vi "Set RX Data Width.vi"(8 "error in":errorcluster, 10 "rx internal data width":T1=enum."32 Bit", 11 "eye scan in":refnum<class "niHighSpeedSerial Eye Scan v1 Host.lvclass">) -> (0 "error out":errorcluster, 3 "eye scan out":refnum<class "niHighSpeedSerial Eye Scan v1 Host.lvclass">)   [LabVIEW 2015, in "niHighSpeedSerial Eye Scan v1 Host.lvclass"]
uses:
  <instrlib>/niHighSpeedSerial/Eye Scan/v1/Host/Eye Scan/niHighSpeedSerial Eye Scan v1 Host.lvclass
  <instrlib>/niHighSpeedSerial/Eye Scan/v1/Host/Common/Public/Data Width.ctl
  <instrlib>/niHighSpeedSerial/Eye Scan/v1/Host/Eye Scan/niHighSpeedSerial Eye Scan v1 Host.lvclass/niHighSpeedSerial Eye Scan v1 Host.ctl
  <vilib>/Utility/error.llb/Error Cluster From Error Code.vi
  <vilib>/ErrorRing/Error Ring.xnode
  <instrlib>/niHighSpeedSerial/Eye Scan/v1/Host/Common/niHighSpeedSerial Eye Scan Common v1 Host.lvlib
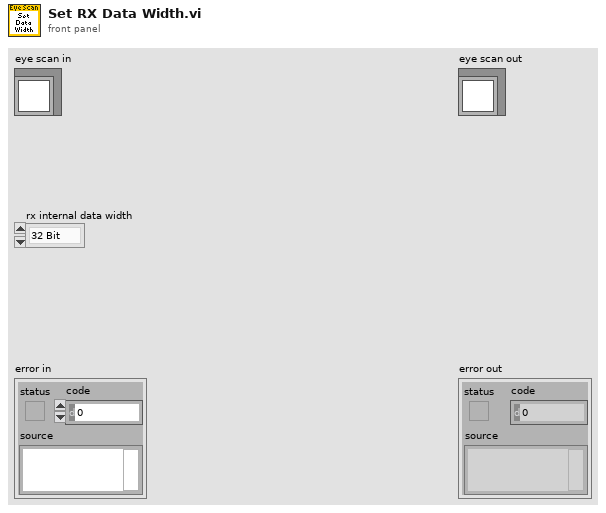
[diagram p1: front panel]
types:
  T1 = typedef "niHighSpeedSerial Eye Scan Common v1 Host.lvlib/Data Width.ctl" = enum16{"16 Bit", "20 Bit", "32 Bit", "40 Bit"}
  T2 = typedef "niHighSpeedSerial Eye Scan v1 Host.lvclass/Private Data.ctl" = cluster{"instruction target":refnum<class "niInstr Instruction Target v1 Host.lvclass">, "channels":T3[], "measure state":T4, "rx output divider":T5, "equalization mode":T6, "rx internal data width":T1, "BER floor":dbl, "number of points completed":i32, "rx output divider configured?":bool, "equalization mode configured?":bool, "rx data width configured?":bool}
  T3 = typedef "niHighSpeedSerial Eye Scan v1 Host.lvclass/Channel Data.ctl" = cluster{"instance":u8, "channel":refnum<class "niHighSpeedSerial Eye Scan Single Point v1 Host.lvclass">, "point iterator":refnum<class "niHighSpeedSerial Eye Scan Point Iterator v1 Host.lvclass">}
  T4 = typedef "niHighSpeedSerial Eye Scan v1 Host.lvclass/Measure State.ctl" = enum16{"Uninitialized", "Initialized", "Ready", "Measuring", "Finished", "Aborted"}
  T5 = typedef "niHighSpeedSerial Eye Scan Common v1 Host.lvlib/RX Output Divider.ctl" = enum16{"1", "2", "4", "8", "16"}
  T6 = typedef "niHighSpeedSerial Eye Scan Common v1 Host.lvlib/Equalization Mode.ctl" = enum16{"DFE", "LPM"}
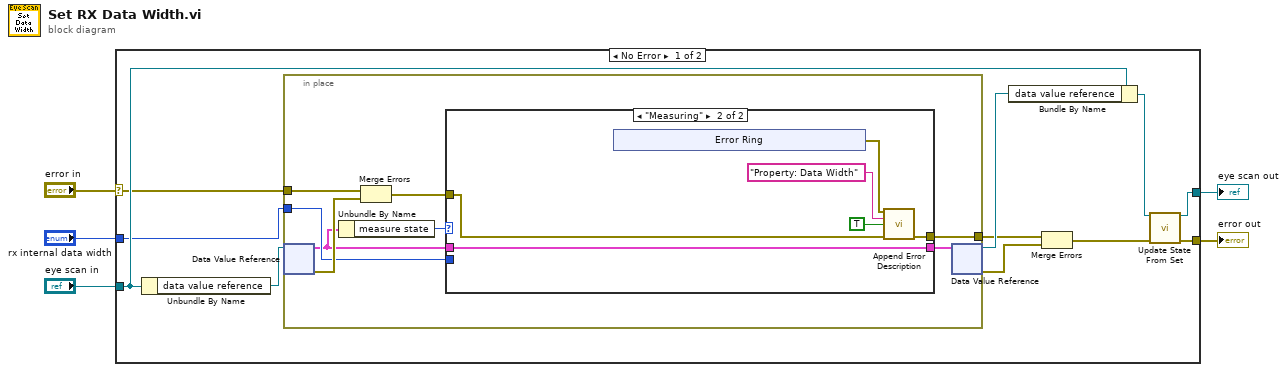
[diagram p0: block diagram]
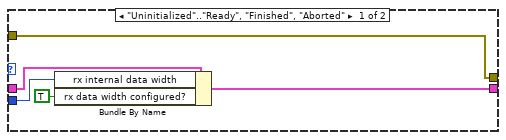
[diagram p2: hidden frame]
diagram:
  n1 = case shown="No Error" "error in" {
    selector: "error in" -> [w13 w41]
    tunnel: [w6 w41] -> w4
    tunnel: [w8 w40] -> w2
    tunnel: "eye scan in" -> [w15 w40]
    tunnel: "rx internal data width" -> [w10 _]
    frame No Error {
      n2 = Unbundle By Name(w15) -> ("data value reference"=w16:refnum<data-value>)
      n3 = in-place {
        in-place-border: w13 -> [w24]
        in-place-border: [w20] -> w11
        in-place-border: w10 -> [w22]
        n4 = in-place-dvr #1(w16) -> (w18:T2, w23:errorcluster)
        n5 = Unbundle By Name(w18) -> ("measure state"=w17:T4)
        n6 = Merge Errors(w24, w23) -> (w21:errorcluster)
        n7 = case shown="\"Measuring\"" w17 {
          tunnel: w21 -> [w29 w32]
          tunnel: [w29 w33] -> w20
          tunnel: w22 -> [w27 _]
          tunnel: w18 -> [w28 w35]
          tunnel: [w26 w35] -> w19
          frame "Uninitialized".."Ready", "Finished", "Aborted" {
            n8 = Bundle By Name(cluster=w28, "rx internal data width"=w27, "rx data width configured?"=TRUE ("data width configured?")) -> (w26:T2)
          }
          frame "Measuring" {
            n9 = xnode "Error Ring"() -> ("error out"=w34:errorcluster)
            n10 = call <instrlib>:"Append Error Description.vi"("error to append"=w34, "append string (\"\")"="Property: Data Width" ("replace string (\"\")"), "generate error?"=TRUE, "error in"=w32) -> ("error out"=w33:errorcluster)  [unwired: 11 in]
          }
        }
        n11 = in-place-dvr #1(w19) -> (w14:refnum<data-value>, w12:errorcluster)
      }
      n12 = Bundle By Name(cluster=w15, "data value reference"=w14) -> (w9:refnum<class "niHighSpeedSerial Eye Scan v1 Host.lvclass">)
      n13 = Merge Errors(w11, w12) -> (w7:errorcluster)
      n14 = call-dynamic "Update State From Set.vi"("eye scan in"=w9, "error in"=w7) -> ("eye scan out"=w8:refnum<class "niHighSpeedSerial Eye Scan v1 Host.lvclass">, "error out"=w6:errorcluster)  [unwired: 12 in]
    }
    frame Error {
    }
  }
  "error out" <- w4
  "eye scan out" <- w2
